vi "Exemple_7.vi"() -> ()   [LabVIEW 2018]
panel:
  out "Produit":i16
  out "N-2":i8
  out "N-1":i8
  out "N":i8
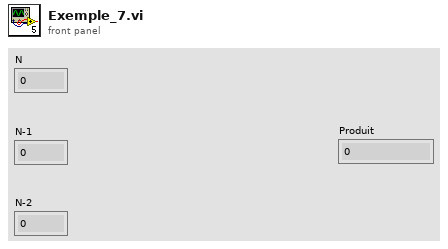
[diagram p1: front panel]
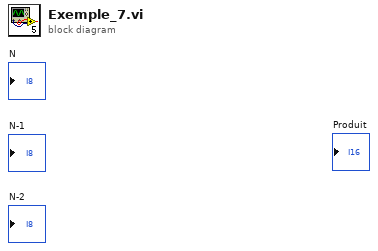
[diagram p0: block diagram]
diagram:
